vi "Read Page Selector Visible.vi"(8 "error in (no error)":errorcluster, 11 "PageSelector.lvclass in":refnum<class "PageSelector.lvclass">) -> (0 "error out":errorcluster, 2 "PageSelVis":bool, 3 "PageSelector.lvclass out":refnum<class "PageSelector.lvclass">)   [LabVIEW 2015, in "PageSelector.lvclass"]
uses:
  PageSelector.lvclass
  PageSelector.lvclass/PageSelector.ctl
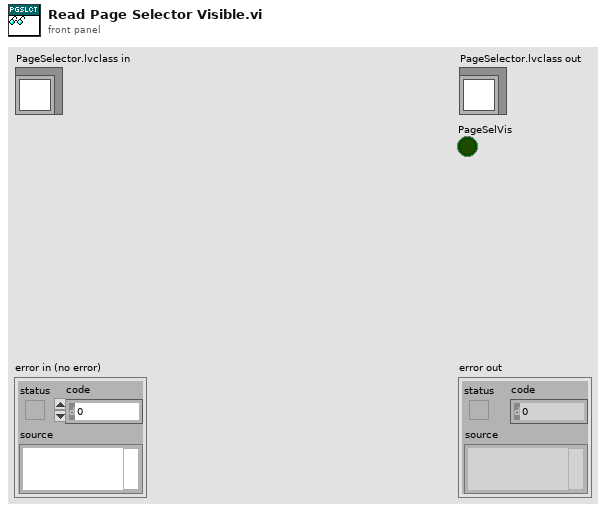
[diagram p1: front panel]
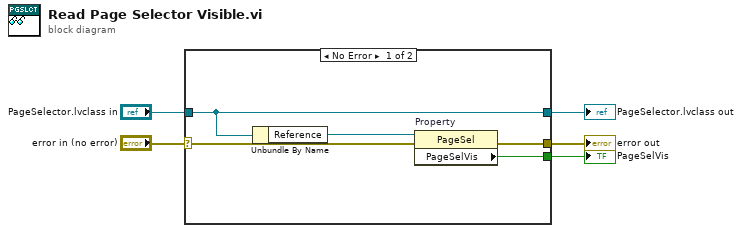
[diagram p0: block diagram]
diagram:
  n1 = case shown="No Error" "error in (no error)" {
    selector: "error in (no error)" -> [w6 w12]
    tunnel: [w9 w12] -> w4
    tunnel: [w8 w11] -> w2
    tunnel: "PageSelector.lvclass in" -> [w8 w11]
    tunnel: [w10 _] -> w1
    frame No Error {
      n2 = Unbundle By Name(w8) -> ("Reference"=w7:refnum<vi>)
      n3 = property on="Property" class="PageSel"(reference=w7, error in=w6) -> (error out=w9:errorcluster, "PageSelVis"=w10:bool)  [unwired: 1 out]
    }
    frame Error {
    }
  }
  "error out" <- w4
  "PageSelector.lvclass out" <- w2
  "PageSelVis" <- w1
